vi "Set Array of Move Button Configurations.vi"(8 "error in (no error)":errorcluster, 10 "Array of Move Button Configurations":T1[](array[typedef]) {"Target pos" format="%#_f mm"}, 11 "VacuumLine Configuration in":refnum<class "VacuumLine Configuration.lvclass">) -> (0 "error out":errorcluster, 3 "VacuumLine Configuration out":refnum<class "VacuumLine Configuration.lvclass">)   [LabVIEW 2016, in "Hardware.lvlib" / "VacuumLine.lvlib" / "VacuumLine Configuration.lvclass"]
uses:
  <userlib>/Common Components/Hardware/Abstract System/VacuumLine/VacuumLine Config/VacuumLine Configuration.lvclass
  <userlib>/Common Components/Hardware/Abstract System/VacuumLine/VacuumLine/Button Config Cluster.ctl
  <userlib>/Common Components/Hardware/Abstract System/VacuumLine/VacuumLine Config/VacuumLine Configuration.lvclass/VacuumLine Configuration.ctl
  <userlib>/Common Components/Hardware/Abstract System/VacuumLine/VacuumLine/VacuumLine.lvclass/VacuumLine.ctl
  <userlib>/Common Components/Hardware/Abstract System/VacuumLine/VacuumLine/VacuumLine.lvclass
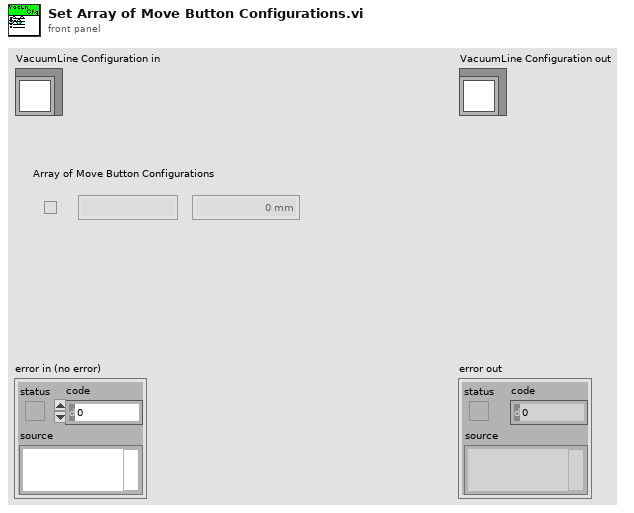
[diagram p1: front panel]
types:
  T1 = typedef "Hardware.lvlib/VacuumLine.lvlib/VacuumLine.lvclass/Button Config Cluster.ctl" = cluster{"Enabled?":bool, "Text on button":string, "Target pos":dbl}
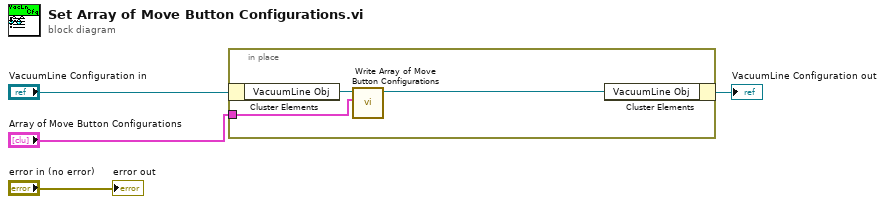
[diagram p0: block diagram]
diagram:
  n1 = in-place {
    in-place-border: "Array of Move Button Configurations" -> [w5]
    n2 = in-place-cluster #1("VacuumLine Configuration in") -> ("VacuumLine Obj"=w7:refnum<class "VacuumLine.lvclass">)
    n3 = call <userlib>:"Write Array of Move Button Configurations.vi"("Array of Move Button Configurations"=w5, "VacuumLine in"=w7) -> ("VacuumLine out"=w6:refnum<class "VacuumLine.lvclass">)  [unwired: 9 in]
    n4 = in-place-cluster #1("VacuumLine Obj"=w6) -> (→"VacuumLine Configuration out":refnum<class "VacuumLine Configuration.lvclass">)
  }
  "error out" <- "error in (no error)"
